vi "save_tdms.vi"(8 "error in (no error)":errorcluster, 10 "Data":dbl[](array[numeric]), 11 "Path":path) -> (0 "error out":errorcluster)   [LabVIEW 2024]
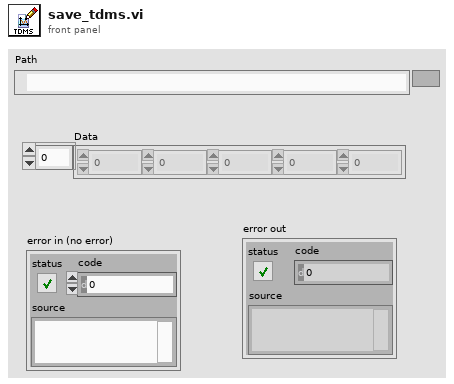
[diagram p1: front panel]
types:
  T1 = enum16{"open", "open or create", "create or replace", "create", "open (read-only)"}
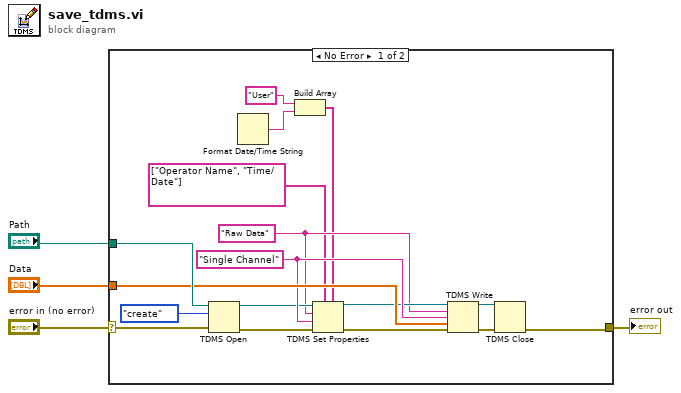
[diagram p0: block diagram]
diagram:
  n1 = case shown="No Error" "error in (no error)" {
    selector: "error in (no error)" -> [w21 w22]
    tunnel: [w17 w22] -> w3
    tunnel: "Path" -> [w15 _]
    tunnel: "Data" -> [w14 _]
    frame No Error {
      w9 = "Raw Data" ("group name in (Untitled)")
      w13 = "Single Channel" ("channel name")
      n2 = TDMS Open(8:w21, 10:T1."create" ("operation (0:open)"), 11:w15) -> (0:w20:errorcluster, 3:w10:refnum<k34>)  [unwired: 4 in]
      n3 = Format Date/Time String() -> (date/time string=w7:string)  [unwired: 3 in]
      n4 = Build Array("User" ("group name in (Untitled)"), w7) -> (w5:string[])
      n5 = TDMS Set Properties(5:w5, 7:string[] ["Operator Name", "Time/Date"] ("property names"), 8:w20, 9:w13, 10:w9, 11:w10) -> (0:w19:errorcluster, 3:w11:refnum<k34>)  [unwired: 2 out]
      n6 = TDMS Write(0:w11, 5:w9, 7:w13, 9:w14, 11:w19) -> (4:w12:refnum<k34>, 15:w18:errorcluster)  [unwired: 1 in, 2 out]
      n7 = TDMS Close(8:w18, 11:w12) -> (0:w17:errorcluster)  [unwired: 1 out]
    }
    frame Error {
    }
  }
  "error out" <- w3
